vi "SystemTestIterator.vi"(8 "error in (no error)":errorcluster) -> (0 "error out":errorcluster, 3 "This VI":refnum<vi>)   [LabVIEW 2018]
uses:
  Test Parameter Globals_1.0.0.vi
  Test Result File Name Global.vi
  <vilib>/Utility/file.llb/Write Delimited Spreadsheet (string).vi
  Initialize References/Sequence Globals.vi
  <vilib>/Utility/file.llb/Read Delimited Spreadsheet (string).vi
  Automated Tests/Tetra WAM/Tetra_Globals.vi
panel:
  in  "prompt on fail(t)":bool
  out "Pass(T)":bool
  out "Revision_Payload":string
  out "Revision_Setup":string
  in  "Pause":bool=TRUE caption="Enable"
  out "Iteration Info":string="0" caption="1607 of 1608 Iterations Remaining..."
  out "Avg Time (s)":dbl
  out "Time Remain":dbl
  out "# of iterations":i32
  out "Parameter                                Result":string[][](array[string])
  out "Current Iteration":i32=1
  out "Result File Name":path
  out "Column Headers Global":string[](array[string])=["CHANNEL", "VCC", "RF_FREQ", "LO_LEVEL", "IF_FREQ", "F_DELTA", "P_IN_RF", "IP3L(dBm)", "IP3H(dBm)", "PoutIF1(dBm)", "PoutIF2(dBm)", "IM3L(dBm)", "IM3H(dBm)", "IP3_MIN(dBm)", "IM2L(dBm)", "IM2H(dBm)", "2x2 Spur(dBm)", "2x2 Spur( -dBc)", "3x3 Spur(dBm)", "3x3 Spur( -dBc)", "Gain F1(dB)", "Pin @1dB(dBm)", "Pout @1dB(dBm)", "LO>IF(dBm)", "RF>IF(dBm)", "ICC(A)", "Pin RF1(dBm corrected)", "Pin RF2(dBm corrected)", "LO Freq(Hz)", "RF1 Freq(Hz)", "RF2 Freq(Hz)", "IF1 Freq(Hz)", "IF2 Freq(Hz)", "NxM Spur1 RF Freq (Hz)", "NxM Spur2 RF Freq (Hz)", "SA Attn Value(dB)"]
  out "Status":string
  out "Payload ref":refnum<vi>
  out "Payload Results":string[](array[string])
  out "Progress":dbl(slide) caption="... Minutes remaim" scale=0.0..100.0
  out "Total Time":dbl=7.28125
  in  "Stop Iterator":bool
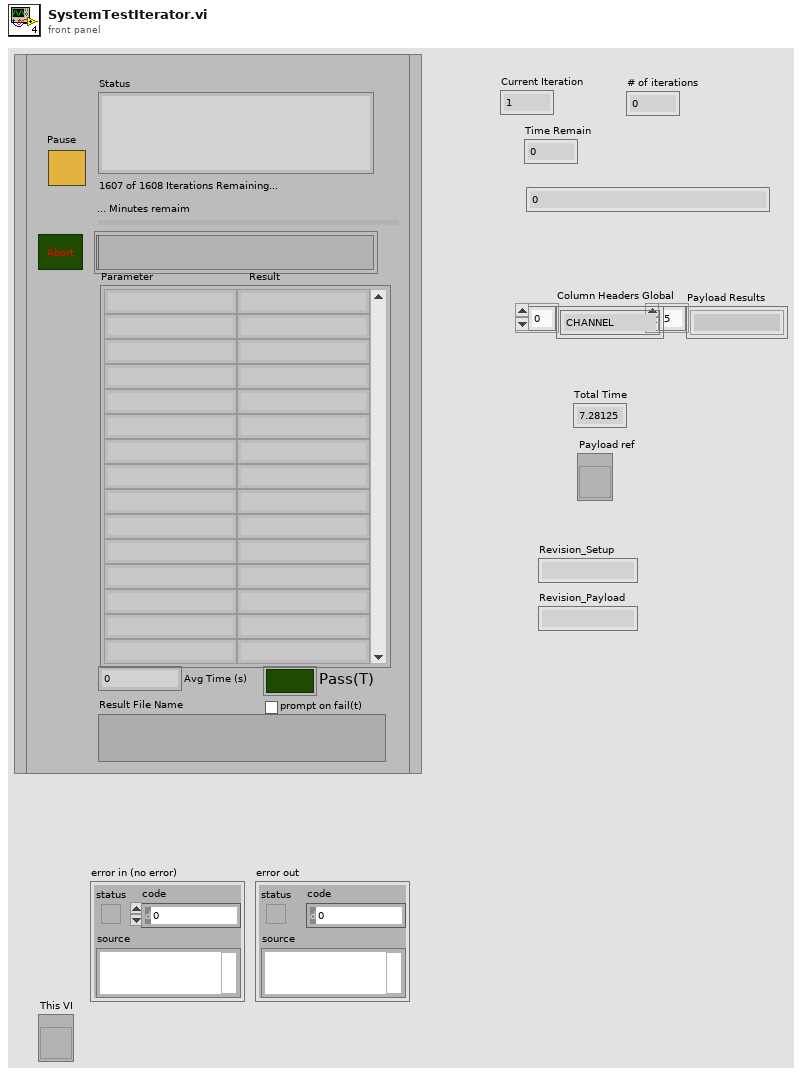
[diagram p1: front panel]
types:
  T1 = enum32{"Invalid", "Standard", "Closed", "Hidden", "Minimized", "Maximized"}
  T2 = enum16{"Left Button", "Center Button", "Right Button", "Window Close"}
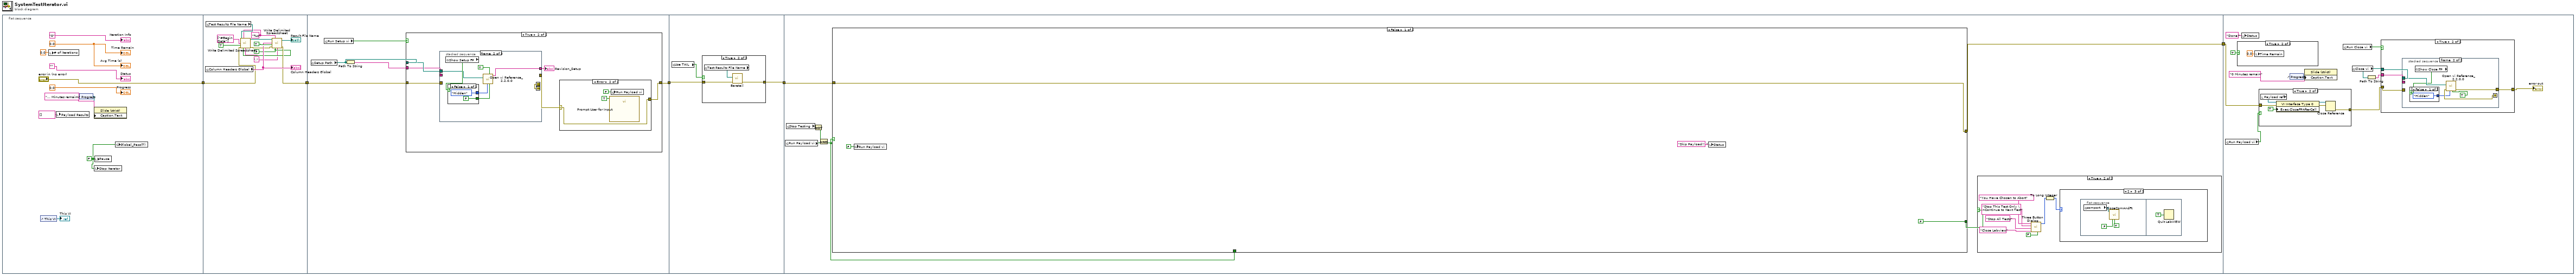
[diagram p0: block diagram]
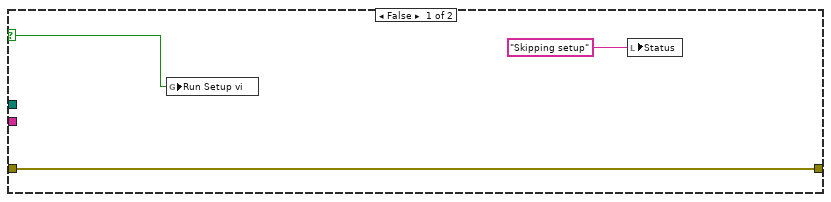
[diagram p2: hidden frame]
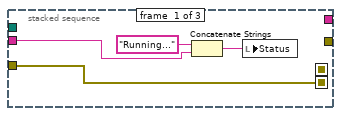
[diagram p4: hidden frame]
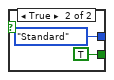
[diagram p5: hidden frame]
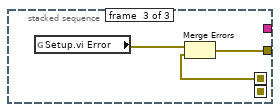
[diagram p6: hidden frame]
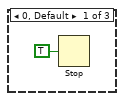
[diagram p9: hidden frame]
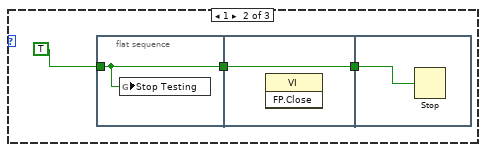
[diagram p10: hidden frame]
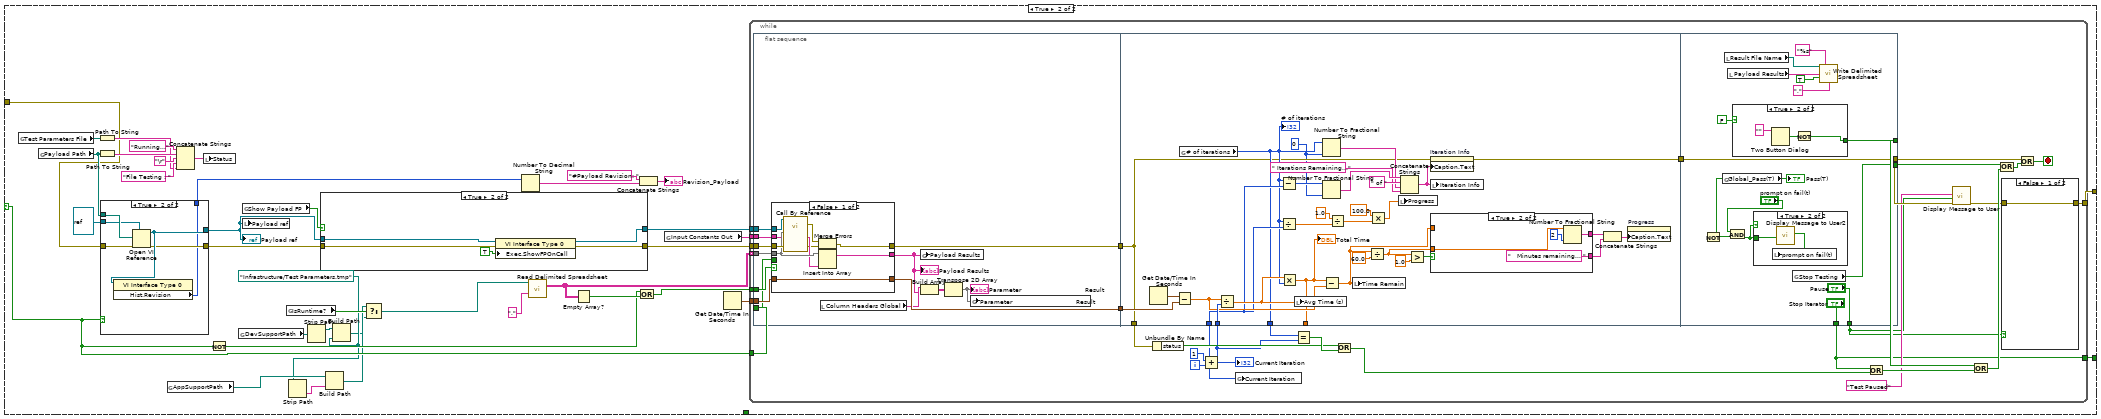
[diagram p11: hidden frame]
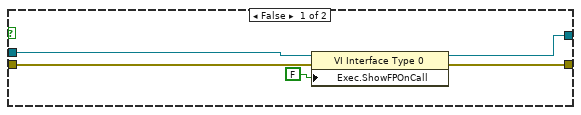
[diagram p12: hidden frame]
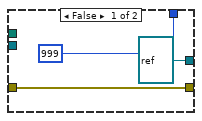
[diagram p13: hidden frame]
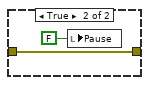
[diagram p14: hidden frame]
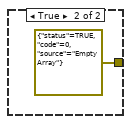
[diagram p16: hidden frame]
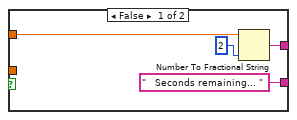
[diagram p17: hidden frame]
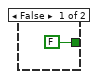
[diagram p19: hidden frame]
diagram:
  n1 = flat-sequence {
    tunnel: ["error in (no error)"] -> w3
    tunnel: [w24] -> w4
    tunnel: w3 -> [w25]
    tunnel: w4 -> [w34]
    tunnel: [w33] -> w2
    tunnel: w2 -> [w68]
    tunnel: [w67] -> w1
    tunnel: [w79] -> w5
    tunnel: w1 -> [w78]
    tunnel: w5 -> [w288]
    frame #0 {
      w7 = FALSE ("Pause")
      w11 = 0.0 ("Time Remain")
      n2 = control-ref of="This VI"() -> (→"This VI":refnum<vi>)
      n3 = local write "# of iterations"(0.0 ("Avg Payload Time (s)")) -> ()
      n4 = local write "Payload Results"(string[] [] ("Payload Results")) -> ()
      n5 = control-ref of="Progress"() -> (w12:refnum<vi>)
      n6 = property on="Property Node" class="Slide (strict)"(reference=w12, "Caption.Text"="... Minutes remaim") -> ()  [unwired: 1 in, 2 out]
      n7 = local write "Stop Iterator"(w7) -> ()
      n8 = local write "Pause"(w7) -> ()
      n9 = global write "Test Parameter Globals_1.0.0.vi" "Global_Pass(T)"(w7) -> ()
      "Status" <- ""
      "Progress" <- 0.0 ("Progress")
      "Time Remain" <- w11
      "Avg Time (s)" <- w11
      "Iteration Info" <- "0" ("Iteration Info")
    }
    frame #1 {
      w17 = "%s" ("format (%s)")
      w23 = FALSE ("transpose? (no:F)")
      w22 = "," ("delimiter (\\t)")
      n10 = global read "Test Parameter Globals_1.0.0.vi" "Column Headers Global"() -> (w28:string[])
      "Column Headers Global" <- w28
      n11 = global read "Test Result File Name Global.vi" "Test Results File Name"() -> (w18:path)
      n12 = call-poly <vilib>:"Write Delimited Spreadsheet.vi"("file path (dialog if empty)"=w18, "format (%s)"=w17, "1D data"=string[] ["#Begin Data"] ("Payload Results"), "append to file? (new file:F)"=TRUE, "error in (no error)"=w25, "transpose? (no:F)"=w23, "delimiter (\\t)"=w22) -> ("new file path (Not A Path if cancelled)"=w19:path, "error out"=w26:errorcluster)  [unwired: 7 in]
      n13 = call-poly <vilib>:"Write Delimited Spreadsheet.vi"("file path (dialog if empty)"=w19, "format (%s)"=w17, "1D data"=w28, "append to file? (new file:F)"=TRUE, "error in (no error)"=w26, "transpose? (no:F)"=w23, "delimiter (\\t)"=w22) -> ("new file path (Not A Path if cancelled)"=→"Result File Name":path, "error out"=w24:errorcluster)  [unwired: 7 in]
    }
    frame #2 {
      n14 = global read "Test Parameter Globals_1.0.0.vi" "Setup Path"() -> (w32:path)
      n15 = global read "Test Parameter Globals_1.0.0.vi" "Run Setup vi"() -> (w31:bool)
      n16 = Path To String(path=w32) -> (string=w30:string)
      n17 = case shown="True" w31 {
        selector: w31 -> [w35 _]
        tunnel: w34 -> [w37 w43]
        tunnel: [w37 w40] -> w33
        tunnel: w32 -> [_ w42]
        tunnel: w30 -> [_ w41]
        frame False {
          n18 = global write "Test Parameter Globals_1.0.0.vi" "Run Setup vi"(w35) -> ()
          n19 = local write "Status"("Skipping setup") -> ()
        }
        frame True {
          n20 = stacked-sequence {
            seq-local: [w48 _ _] -> [_ w53 _]
            seq-local: [_ w53 _] -> [_ _ w64]
            tunnel: w43 -> [w48 _ _]
            tunnel: w42 -> [_ w55 _]
            tunnel: w41 -> [w49 _ _]
            tunnel: [_ _ w63] -> w39
            tunnel: [_ w54 _] -> w38
            frame #0 {
              n21 = Concatenate Strings("Running..." ("string"), w49) -> (w51:string)
              n22 = local write "Status"(w51) -> ()
            }
            frame #1 {
              n23 = global read "Test Parameter Globals_1.0.0.vi" "Show Setup FP"() -> (w57:bool)
              n24 = case shown="False" w57 {
                tunnel: [T1."Hidden" ("Front Panel State") T1."Standard" ("Front Panel State")] -> w58
                tunnel: [FALSE ("Close vi") TRUE ("Close vi")] -> w52
                frame False {
                }
                frame True {
                }
              }
              n25 = call "Open vi Reference_2.2.0.0.vi"("Close Front Panel(T)"=w52, "Wait Until Done"=TRUE, "Front Panel State"=w58, "vi path"=w55) -> ("hist_rev"=w54:string)  [unwired: 4 in, 3 out]
            }
            frame #2 {
              n26 = global read "Test Parameter Globals_1.0.0.vi" "Setup.vi Error"() -> (w65:errorcluster)
              n27 = Merge Errors(w65, w64) -> (w63:errorcluster)
            }
          }
          "Revision_Setup" <- w38
          n28 = case shown="Error" w39 {
            selector: w39 -> [w44 w45]
            tunnel: [w44 w45] -> w40
            frame No Error {
            }
            frame Error {
              n29 = call "Prompt User for Input"("Enable"=TRUE) -> ()  [unwired: 17 in, 2 out]
              n30 = global write "Test Parameter Globals_1.0.0.vi" "Run Payload vi"(FALSE ("Run Payload vi")) -> ()
            }
          }
        }
      }
    }
    frame #3 {
      n31 = global read "Test Parameter Globals_1.0.0.vi" "Use TAIL"() -> (w66:bool)
      n32 = case shown="True" w66 {
        tunnel: w68 -> [w69 w71]
        tunnel: [w69 w70] -> w67
        frame False {
        }
        frame True {
          n33 = global read "Test Result File Name Global.vi" "Test Results File Name"() -> (w72:path)
          n34 = call "Baretail.vi"("error in (no error)"=w71, "PATH"=w72) -> ("error out"=w70:errorcluster)  [unwired: 8 in, 1 out]
        }
      }
    }
    frame #4 {
      n35 = global read "Test Parameter Globals_1.0.0.vi" "Run Payload vi"() -> (w73:bool)
      n36 = global read "Sequence Globals.vi" "Stop Testing"() -> (w74:bool)
      n37 = Not(x=w74) -> (.not. x?=w76:bool)
      n38 = And(x=w76, y=w73) -> (x .and. y?=w75:bool)
      n39 = case shown="False" w75 {
        selector: w75 -> [_ w112]
        tunnel: [FALSE ("Stop Iterator") w138] -> w77
        tunnel: [w99 w137] -> w79
        tunnel: w75 -> [_ _]
        tunnel: w78 -> [w99 w106]
        frame False {
          n40 = global write "Test Parameter Globals_1.0.0.vi" "Run Payload vi"(FALSE ("Run Payload vi")) -> ()
          n41 = local write "Status"("Skip Payload!!  " ("Status")) -> ()
        }
        frame True {
          w103 = path "Infrastructure/Test Parameters.tmp" ("file path (dialog if empty)")
          n42 = global read "Test Parameter Globals_1.0.0.vi" "Test Parameters File"() -> (w123:path)
          n43 = global read "Test Parameter Globals_1.0.0.vi" "Payload Path"() -> (w132:path)
          n44 = Path To String(path=w123) -> (string=w120:string)
          n45 = Path To String(path=w132) -> (string=w135:string)
          n46 = case shown="True" w112 {
            tunnel: w132 -> [_ w158]
            tunnel: refnum<vi> refnum ("type specifier VI Refnum (for type only)") -> [_ w157]
            tunnel: [refnum<vi> refnum ("type specifier VI Refnum (for type only)") w156] -> w114
            tunnel: [w151 w155] -> w119
            tunnel: w106 -> [w151 w154]
            tunnel: [u32 999 ("Hist.Revision") w153] -> w113
            frame False {
            }
            frame True {
              n47 = Open VI Reference(type specifier VI Refnum (for type only)=w157, vi path=w158, error in (no error)=w154) -> (vi reference=w156:refnum<vi>, error out=w155:errorcluster)  [unwired: 3 in]
              n48 = property class="VI Interface Type 0"(reference=w156) -> ("Hist.Revision"=w153:u32)  [unwired: 1 in, 2 out]
            }
          }
          "Payload ref" <- w114
          n49 = global read "Sequence Globals.vi" "AppSupportPath"() -> (w108:path)
          n50 = Concatenate Strings("Running..." ("string"), w135, "\r", "File Testing : " ("string"), w120) -> (w133:string)
          n51 = local write "Status"(w133) -> ()
          n52 = Not(x=w112) -> (.not. x?=w127:bool)
          n53 = global read "Sequence Globals.vi" "DevSupportPath"() -> (w105:path)
          n54 = global read "Test Parameter Globals_1.0.0.vi" "Show Payload FP"() -> (w124:bool)
          n55 = local write "Payload ref"(w114) -> ()
          n56 = global read "Sequence Globals.vi" "IsRuntime?"() -> (w111:bool)
          n57 = Strip Path(path=w103) -> (name=w109:string)  [unwired: 1 out]
          n58 = Strip Path(path=w105) -> (stripped path=w104:path)  [unwired: 1 out]
          n59 = case shown="True" w124 {
            tunnel: [w144 w149] -> w130
            tunnel: w114 -> [w143 w148]
            tunnel: [w142 w147] -> w129
            tunnel: w119 -> [w141 w146]
            frame False {
              n60 = property class="VI Interface Type 0"(reference=w143, error in=w141, "Exec.ShowFPOnCall"=FALSE ("Execution:Show Front Panel On Call")) -> (reference out=w144:refnum<vi>, error out=w142:errorcluster)
            }
            frame True {
              n61 = property class="VI Interface Type 0"(reference=w148, error in=w146, "Exec.ShowFPOnCall"=TRUE ("Execution:Show Front Panel On Call")) -> (reference out=w149:refnum<vi>, error out=w147:errorcluster)
            }
          }
          n62 = Build Path(base path=w108, name or relative path=w109) -> (appended path=w107:path)
          n63 = Build Path(base path=w104, name or relative path=w103) -> (appended path=w102:path)
          n64 = Select(t=w107, s=w111, f=w102) -> (s? t:f=w110:path)
          n65 = Number To Decimal String(number=w113) -> (decimal integer string=w117:string)  [unwired: 1 in]
          n66 = call-poly <vilib>:"Read Delimited Spreadsheet.vi"("file path (dialog if empty)"=w110, "delimiter (\\t)"="," ("delimiter (\\t)")) -> ("all rows"=w125:string[][])  [unwired: 8 in, 5 out]
          n67 = Empty Array?(array=w125) -> (empty?=w136:bool)
          n68 = Or(x=w127, y=w136) -> (x .or. y?=w128:bool)
          n69 = Concatenate Strings("#Payload Revision: " ("string"), w117) -> (→"Revision_Payload":string)
          n70 = global read "Test Parameter Globals_1.0.0.vi" "Input Constants Out"() -> (w131:string[])
          n71 = Get Date/Time In Seconds() -> (seconds since 1Jan1904=w139:timestamp)
          n72 = while {
            tunnel: w125 -> [w187] mode=indexing
            tunnel: w139 -> [w181]
            tunnel: [w159] -> w138
            tunnel: [w162] -> w137
            tunnel: w128 -> [w176]
            tunnel: w130 -> [w172]
            tunnel: w129 -> [w171]
            tunnel: w131 -> [w170]
            tunnel: w112 -> [w169]
            i -> [w186]
            stop <- w166 stop-if-true
            n73 = flat-sequence {
              tunnel: w187 -> [w204]
              tunnel: w181 -> [w202]
              tunnel: [w203] -> w179
              tunnel: [w192] -> w178
              tunnel: w176 -> [w201]
              tunnel: w172 -> [w200]
              tunnel: w171 -> [w193]
              tunnel: w170 -> [w199]
              tunnel: w169 -> [w196]
              tunnel: w168 -> [w249]
              tunnel: [w227] -> w184
              tunnel: w168 -> [w231]
              tunnel: [w241] -> _
              tunnel: w179 -> [w243]
              tunnel: w178 -> [w223]
              tunnel: [w222] -> w177
              tunnel: [w223] -> w173
              tunnel: [w272] -> w182
              tunnel: [w271] -> w165
              tunnel: w177 -> [w271]
              tunnel: [w261] -> w161
              tunnel: ["Pause"] -> w160
              tunnel: ["Stop Iterator"] -> w159
              frame #0 {
                n74 = case shown="False" w201 {
                  tunnel: w204 -> [w210 _]
                  tunnel: [w214 w218] -> w203
                  tunnel: w202 -> [w214 w218]
                  tunnel: [w205 w217] -> w192
                  tunnel: w200 -> [w213 _]
                  tunnel: [w211 _] -> w194
                  tunnel: w193 -> [w212 w216]
                  tunnel: w199 -> [w208 _]
                  tunnel: w196 -> [_ w215]
                  frame False {
                    n75 = call-by-ref "?"(reference=w213, "error in (no error)"=w212, "Input Constants"=w208, "Parameters"=w210) -> (error out=w207:errorcluster, 0:"error out"=w206:errorcluster, "Payload Results"=w209:string[])  [unwired: 8 in, 1 out]
                    n76 = Merge Errors(w207, w206) -> (w205:errorcluster)
                    n77 = Insert Into Array(array=w210, new element=w209) -> (w211:string[])  [unwired: 1 in]
                  }
                  frame True {
                    n78 = case shown="False" w215 {
                      tunnel: [w219 errorcluster {"status"=TRUE, "code"=0, "source"="Empty Array"} ("error out")] -> w217
                      tunnel: w216 -> [w219 _]
                      frame False {
                      }
                      frame True {
                      }
                    }
                  }
                }
                "Payload Results" <- w194
                n79 = local read "Column Headers Global"() -> (w198:string[])
                n80 = global write "Test Parameter Globals_1.0.0.vi" "Payload Results"(w194) -> ()
                n81 = Build Array(w198, w194) -> (w197:string[][])
                n82 = Transpose 2D Array(2D array=w197) -> (transposed array=w195:string[][])
                "Parameter                                Result" <- w195
                n83 = global write "Test Parameter Globals_1.0.0.vi" "Parameter                                Result"(w195) -> ()
              }
              frame #1 {
                w221 = i16 0 ("precision (6)")
                n84 = Get Date/Time In Seconds() -> (seconds since 1Jan1904=w250:timestamp)
                n85 = Subtract(x=w250, y=w243) -> (x-y=w244:dbl)
                n86 = global read "Test Parameter Globals_1.0.0.vi" "# of iterations"() -> (w227:i32)
                "# of iterations" <- w227
                n87 = Divide(x=w244, y=w249) -> (x/y=w233:dbl)
                n88 = Subtract(x=w227, y=w231) -> (x-y=w230:i32)
                n89 = Divide(x=w227, y=w231) -> (x/y=w247:dbl)
                n90 = Multiply(x=w233, y=w227) -> (x*y=w241:dbl)
                "Total Time" <- w241
                n91 = local write "Avg Time (s)"(w233) -> ()
                n92 = Number To Fractional String(number=w227, precision (6)=w221) -> (F-format string=w226:string)  [unwired: 2 in]
                n93 = Number To Fractional String(number=w230, precision (6)=w221) -> (F-format string=w229:string)  [unwired: 2 in]
                n94 = Subtract(x=w241, y=w244) -> (x-y=w232:dbl)
                n95 = Divide(x=1.0, y=w247) -> (x/y=w246:dbl)
                n96 = local write "Time Remain"(w232) -> ()
                n97 = Divide(x=w232, y=60.0) -> (x/y=w236:dbl)
                n98 = Multiply(x=100.0, y=w246) -> (x*y=w234:dbl)
                n99 = local write "Progress"(w234) -> ()
                n100 = Concatenate Strings(w229, " of " ("string"), w226, " Iterations Remaining..." ("string")) -> (w224:string)
                n101 = Greater?(x=w236, y=1.0) -> (0:w237:bool)
                n102 = property on="Iteration Info" class="Str"(error in=w223, "Caption.Text"=w224) -> (error out=w222:errorcluster)  [unwired: 1 in, 1 out]
                n103 = local write "Iteration Info"(w224) -> ()
                n104 = case shown="True" w237 {
                  tunnel: [w254 w257] -> w240
                  tunnel: ["   Seconds remaining... " ("string") "   Minutes remaining... " ("string")] -> w238
                  tunnel: w236 -> [_ w255]
                  tunnel: w232 -> [w251 _]
                  frame False {
                    n105 = Number To Fractional String(number=w251, precision (6)=i16 2) -> (F-format string=w254:string)  [unwired: 2 in]
                  }
                  frame True {
                    n106 = Number To Fractional String(number=w255, precision (6)=i16 2) -> (F-format string=w257:string)  [unwired: 2 in]
                  }
                }
                n107 = Concatenate Strings(w240, w238) -> (w239:string)
                n108 = property on="Progress" class="Slide (strict)"("Caption.Text"=w239) -> ()  [unwired: 2 in, 2 out]
              }
              frame #2 {
                n109 = global read "Test Parameter Globals_1.0.0.vi" "Global_Pass(T)"() -> (w264:bool)
                "Pass(T)" <- w264
                n110 = Not(x=w264) -> (.not. x?=w265:bool)
                n111 = local read "Result File Name"() -> (w267:path)
                n112 = local read "Payload Results"() -> (w269:string[])
                n113 = And(x="prompt on fail(t)", y=w265) -> (x .and. y?=w262:bool)
                n114 = case shown="True" FALSE {
                  tunnel: [FALSE ("T button?") w277] -> w272
                  frame False {
                  }
                  frame True {
                    n115 = Two Button Dialog(message="") -> (T button?=w278:bool)  [unwired: 2 in]
                    n116 = Not(x=w278) -> (.not. x?=w277:bool)
                  }
                }
                n117 = case shown="True" w262 {
                  tunnel: w262 -> [_ w275]
                  frame False {
                  }
                  frame True {
                    n118 = call "Display Message to User2"("Enable"=w275) -> ("OK"=w274:bool)  [unwired: 9 in, 1 out]
                    n119 = local write "prompt on fail(t)"(w274) -> ()
                  }
                }
                n120 = global read "Sequence Globals.vi" "Stop Testing"() -> (w261:bool)
                n121 = call-poly <vilib>:"Write Delimited Spreadsheet.vi"("file path (dialog if empty)"=w267, "format (%s)"="%s", "1D data"=w269, "append to file? (new file:F)"=TRUE, "delimiter (\\t)"="," ("delimiter (\\t)")) -> ()  [unwired: 9 in, 2 out]
              }
            }
            n122 = Unbundle By Name(w173) -> ("status"=w174:bool)
            n123 = Add(x=1, y=w186) -> (x+y=w168:i32)
            "Current Iteration" <- w168
            n124 = global write "Sequence Globals.vi" "Current Iteration"(w168) -> ()
            n125 = Equal?(x=w184, y=w168) -> (x = y?=w185:bool)
            n126 = Or(x=w174, y=w185) -> (x .or. y?=w175:bool)
            n127 = Or(x=w159, y=w175) -> (x .or. y?=w183:bool)
            n128 = call "Display Message to User"("error in (no error)"=w165, "Enable"=w160, "Message"="Test Paused") -> ("error out"=w163:errorcluster)  [unwired: 7 in, 1 out]
            n129 = Or(x=w182, y=w183) -> (x .or. y?=w180:bool)
            n130 = Or(x=w161, y=w180) -> (x .or. y?=w167:bool)
            n131 = case shown="False" w160 {
              tunnel: w163 -> [w189 w190]
              tunnel: [w189 w190] -> w162
              frame False {
              }
              frame True {
                n132 = local write "Pause"(FALSE ("Pause")) -> ()
              }
            }
            n133 = Or(x=w165, y=w167) -> (x .or. y?=w166:bool)
          }
        }
      }
      n134 = case shown="True" w77 {
        frame False {
        }
        frame True {
          n135 = call <vilib>:"Three Button Dialog.vi"("Allow user to close window? (TRUE)"=FALSE, "Right Button Text (\"Cancel\")"="Close Labview" ("Right Button Text (\"Cancel\")"), "Center Button Text (\"No\")"="Stop All Tests" ("Center Button Text (\"No\")"), "Left Button Text (\"Yes\")"="Stop This Test Only \nContinue to Next Test" ("Left Button Text (\"Yes\")"), "message"="You Have Chosen to Abort") -> ("Which Button?"=w80:T2)  [unwired: 6 in]
          n136 = To Long Integer(number=w80) -> (32bit integer=w81:i32)
          n137 = case shown="2" w81 {
            frame 0, Default {
              n138 = Stop(stop? (T)=TRUE) -> ()
            }
            frame 1 {
              n139 = flat-sequence {
                tunnel: TRUE ("Stop Testing") -> [w91]
                tunnel: [w91] -> w89
                tunnel: w89 -> [w92]
                tunnel: [w92] -> w88
                tunnel: w88 -> [w93]
                frame #0 {
                  n140 = global write "Sequence Globals.vi" "Stop Testing"(w91) -> ()
                }
                frame #1 {
                  n141 = invoke class="VI" method="FP.Close"() -> ()  [unwired: 3 in, 3 out]
                }
                frame #2 {
                  n142 = Stop(stop? (T)=w93) -> ()
                }
              }
            }
            frame 2 {
              n143 = flat-sequence {
                frame #0 {
                  n144 = global read "Tetra_Globals.vi" "comport"() -> (w94:refnum<visa-resource-name>)
                  n145 = call "CloseComAndFt.vi"("ComPort"=w94, "Skip(T)"=FALSE, "KillFT(t)"=TRUE) -> ()  [unwired: 11 in, 2 out]
                }
                frame #1 {
                  n146 = Quit LabVIEW(quit? (T)=TRUE ("Stop Testing")) -> ()
                }
              }
            }
          }
        }
      }
    }
    frame #5 {
      n147 = global read "Test Parameter Globals_1.0.0.vi" "Run Payload vi"() -> (w280:bool)
      n148 = case shown="True" TRUE {
        frame False {
        }
        frame True {
          n149 = local write "Time Remain"(0.0 ("Time Remain")) -> ()
        }
      }
      n150 = local write "Status"("Done!" ("Status")) -> ()
      n151 = case shown="True" w280 {
        tunnel: w288 -> [w291 w295]
        tunnel: [w291 w294] -> w284
        frame False {
        }
        frame True {
          n152 = local read "Payload ref"() -> (w292:refnum<vi>)
          n153 = property class="VI Interface Type 0"(reference=w292, error in=w295, "Exec.CloseFPAfterCall"=TRUE ("Execution:Close After Call")) -> (reference out=w296:refnum<vi>, error out=w297:errorcluster)
          n154 = Close Reference(reference=w296, error in (no error)=w297) -> (error out=w294:errorcluster)
        }
      }
      n155 = control-ref of="Progress"() -> (w287:refnum<vi>)
      n156 = property on="Property Node" class="Slide (strict)"(reference=w287, "Caption.Text"="0 Minutes remain") -> ()  [unwired: 1 in, 2 out]
      n157 = global read "Test Parameter Globals_1.0.0.vi" "Run Close vi"() -> (w281:bool)
      n158 = global read "Test Parameter Globals_1.0.0.vi" "Close vi"() -> (w282:path)
      n159 = Path To String(path=w282) -> (string=w283:string)
      n160 = case shown="True" w281 {
        tunnel: w284 -> [w299 w303]
        tunnel: [w299 w302] -> w285
        tunnel: w282 -> [_ w301]
        tunnel: w283 -> [_ w300]
        frame False {
          n161 = local write "Status"("Skipping setup") -> ()
        }
        frame True {
          n162 = stacked-sequence {
            seq-local: [w304 _] -> [_ w310]
            tunnel: w303 -> [w304 _]
            tunnel: [_ w312] -> w302
            tunnel: w301 -> [_ w311]
            tunnel: w300 -> [w305 _]
            frame #0 {
              n163 = Concatenate Strings("Running..." ("string"), w305) -> (w307:string)
              n164 = local write "Status"(w307) -> ()
            }
            frame #1 {
              n165 = global read "Test Parameter Globals_1.0.0.vi" "Show Close FP"() -> (w309:bool)
              n166 = case shown="False" w309 {
                tunnel: [T1."Hidden" ("Front Panel State") T1."Standard" ("Front Panel State")] -> w308
                frame False {
                }
                frame True {
                }
              }
              n167 = call "Open vi Reference_2.2.0.0.vi"("Close Front Panel(T)"=TRUE ("Close vi"), "Front Panel State"=w308, "error in"=w310, "vi path"=w311) -> ("error out"=w312:errorcluster)  [unwired: 4 in, 3 out]
            }
          }
        }
      }
      "error out" <- w285
    }
  }
